vi "Launch Dynamic Filter Window.vi"(8 "error in (no error)":errorcluster, 11 "Main Display in":refnum<class "Main Display.lvclass">) -> (0 "error out":errorcluster, 3 "Main Display out":refnum<class "Main Display.lvclass">)   [LabVIEW 2018, in "Assert API Components.lvlib" / "Assert Display.lvlib" / "Main Display.lvlib" / "Main Display.lvclass"]
doc: "Launches the dynamic filter window. Should only ever launch a single instance, further attempts to launch should refer to the same window."
uses:
  Main Display.lvclass
  C:/Program Files (x86)/National Instruments/LabVIEW 2018/vi.lib/ActorFramework/Actor/Actor.lvclass
  Dynamic Filter Window/Dynamic Filter Window/Dynamic Filter Window.lvclass
  Main Display.lvclass/Main Display.ctl
  <vilib>/ActorFramework/Actor/Actor.lvclass
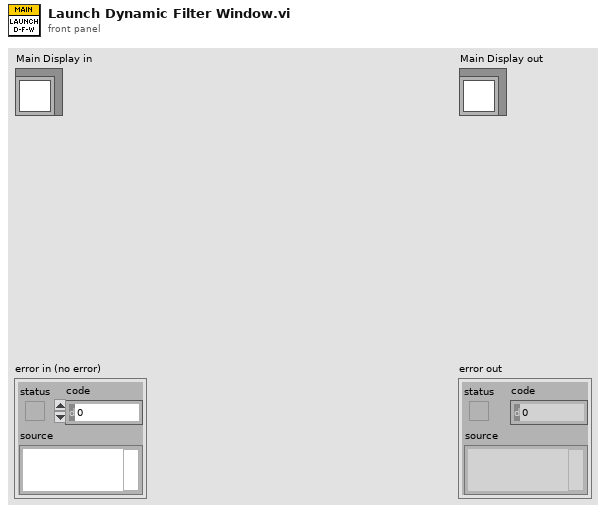
[diagram p1: front panel]
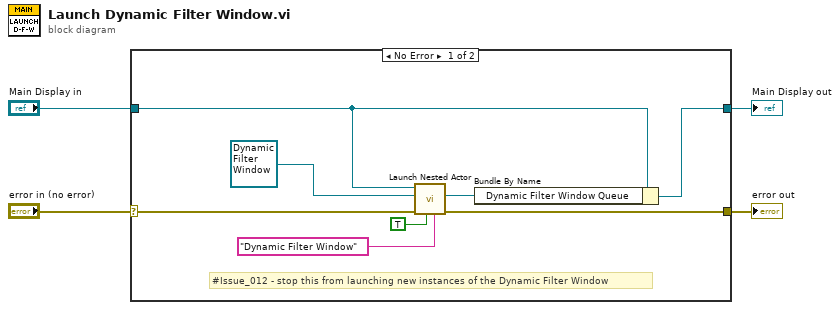
[diagram p0: block diagram]
diagram:
  n1 = case shown="No Error" "error in (no error)" {
    selector: "error in (no error)" -> [w12 w14]
    tunnel: [w11 w14] -> w3
    tunnel: [w8 w13] -> w1
    tunnel: "Main Display in" -> [w10 w13]
    frame No Error {
      # "#Issue_012 - stop this from launching new instances of the Dynamic Filter Window"
      n2 = call <vilib>:"Launch Nested Actor.vi"("Debug Alias"="Dynamic Filter Window", "Open Actor Core front panel? (F)"=TRUE, "error in (no error)"=w12, "Nested Actor"=refnum<class "Dynamic Filter Window.lvclass"> refnum ("Assert API Components.lvlib:Assert Display.lvlib:Main Display.lvlib:Dynamic Filter Window.lvlib:Dynamic Filter Window.lvclass"), "Caller Actor in"=w10) -> ("error out"=w11:errorcluster, "Nested Actor's Enqueuer"=w7:refnum<class "Message Enqueuer.lvclass">)  [unwired: 4 in, 1 out]
      n3 = Bundle By Name(cluster=w10, "Dynamic Filter Window Queue"=w7) -> (w8:refnum<class "Main Display.lvclass">)
    }
    frame Error {
    }
  }
  "error out" <- w3
  "Main Display out" <- w1
